vi "Configure Measurement (TOI - Zero Span).vi"(0 "VISA resource name":refnum<visa-resource-name>, 1 "Auto Zero-Span RBW (T: Enable)":bool=TRUE, 2 "Manual Zero-Span RBW (3E+6 Hz)":dbl=3000000.0, 5 "Enable Zero Span (F: Disable)":bool, 11 "error in (no error)":errorcluster, 12 "Auto Dwell Time (T: Enable)":bool=TRUE, 13 "Dwell Time (1 s)":dbl=1.0) -> (4 "VISA resource name out":refnum<visa-resource-name>, 15 "error out":errorcluster)   [LabVIEW 2014, in "Agilent MXA Series.lvlib"]
doc: "Sets the TOI zero span measurement parameters."
uses:
  Agilent MXA Series.lvlib
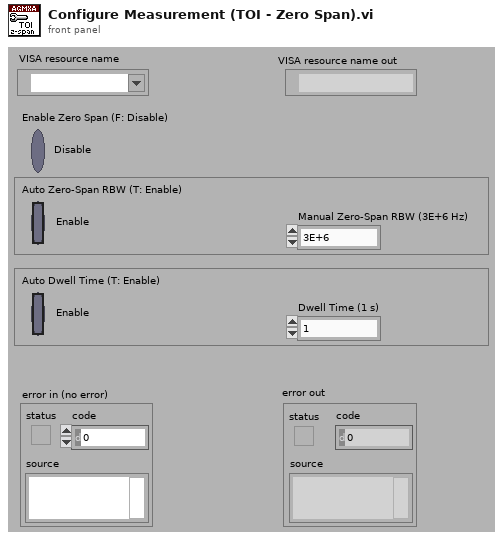
[diagram p1: front panel]
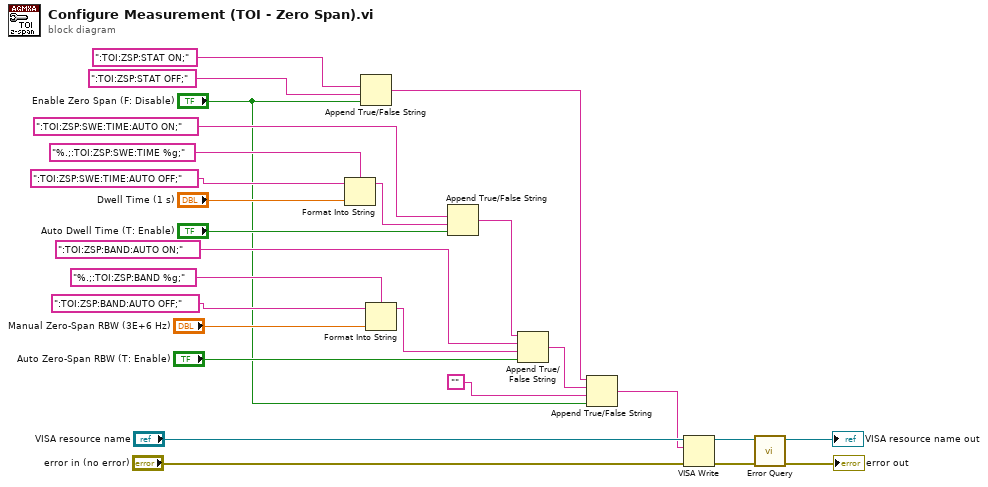
[diagram p0: block diagram]
diagram:
  n1 = Format Into String(format string="%.;:TOI:ZSP:SWE:TIME %g;", initial string=":TOI:ZSP:SWE:TIME:AUTO OFF;", "Dwell Time (1 s)") -> (resulting string=w15:string)  [unwired: 1 in, 1 out]
  n2 = Append True/False String(1:"Enable Zero Span (F: Disable)", 2:":TOI:ZSP:STAT OFF;" ("true string"), 3:":TOI:ZSP:STAT ON;" ("true string")) -> (0:w2:string)  [unwired: 1 in]
  n3 = Format Into String(format string="%.;:TOI:ZSP:BAND %g;", initial string=":TOI:ZSP:BAND:AUTO OFF;", "Manual Zero-Span RBW (3E+6 Hz)") -> (resulting string=w7:string)  [unwired: 1 in, 1 out]
  n4 = Append True/False String(1:"Auto Dwell Time (T: Enable)", 2:w15, 3:":TOI:ZSP:SWE:TIME:AUTO ON;" ("true string")) -> (0:w9:string)  [unwired: 1 in]
  n5 = Append True/False String(1:"Auto Zero-Span RBW (T: Enable)", 2:w7, 3:":TOI:ZSP:BAND:AUTO ON;" ("initial string"), 4:w9) -> (0:w4:string)
  n6 = Append True/False String(1:"Enable Zero Span (F: Disable)", 2:"", 3:w4, 4:w2) -> (0:w3:string)
  n7 = VISA Write(VISA resource name="VISA resource name", write buffer=w3, error in (no error)="error in (no error)") -> (VISA resource name out=w23:refnum<visa-resource-name>, error out=w24:errorcluster)  [unwired: 1 out]
  n8 = call "Error Query.vi"("error in (no error)"=w24, "VISA resource name"=w23) -> ("error out"=→"error out":errorcluster, "VISA resource name out"=→"VISA resource name out":refnum<visa-resource-name>)  [unwired: 6 in, 2 out]
